vi "Map Project TI Name to TS Name.vi"(8 "project targetitem name":string) -> (0 "target structure name":string)   [LabVIEW 2020, in "NI_TargetHelper.lvlib"]
uses:
  <vilib>/TargetSupport/NI_TargetHelper/NI_TargetHelper.lvlib
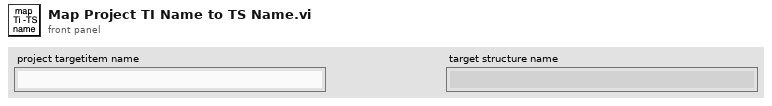
[diagram p1: front panel]
types:
  T1 = cluster{"name":string, "owner":bool, "none":bool, "one":bool, "auto":bool, "choose":bool, "opt#":bool, "ipaddr":bool, "[loc,]mod":bool, "TSname":string}[]
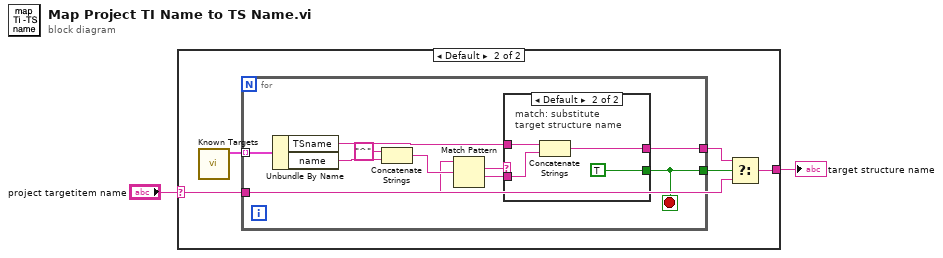
[diagram p0: block diagram]
diagram:
  n1 = case shown="Default" "project targetitem name" {
    selector: "project targetitem name" -> [_ w3]
    tunnel: [_ w4] -> w2
    frame "" {
    }
    frame Default {
      n2 = call <vilib>:"Known Targets.vi"() -> ("targets        project targetItem name              menu to use                    fpga sub                                           suffix info"=w7:T1)  [unwired: 11 in]
      n3 = for {
        tunnel: w7 -> [w17] mode=indexing
        tunnel: w3 -> [w14]
        tunnel: [w10] -> w6
        tunnel: [w9] -> w5
        stop <- w9 stop-if-true
        n4 = Unbundle By Name(w17) -> ("TSname"=w11:string, "name"=w8:string)
        n5 = Concatenate Strings("^" ("string"), w8) -> (w15:string)
        n6 = Match Pattern(string=w14, regular expression=w15) -> (match substring=w13:string, after substring=w12:string)  [unwired: 1 in, 2 out]
        n7 = case shown="Default" w13 {
          tunnel: w12 -> [_ w20]
          tunnel: w11 -> [_ w21]
          tunnel: [_ w19] -> w10
          tunnel: [_ TRUE] -> w9
          frame "" {
            # "no match"
          }
          frame Default {
            # "match: substitute\ntarget structure name"
            n8 = Concatenate Strings(w21, w20) -> (w19:string)
          }
        }
      }
      n9 = Select(t=w6, s=w5, f=w3) -> (s? t:f=w4:string)
    }
  }
  "target structure name" <- w2
